vi "PumpCommand.vi"() -> ()   [LabVIEW 2022 SP3]
panel:
  in  "stop":bool
  in  "reference":refnum<visa-resource-name>
  in  "error in (no error)":errorcluster
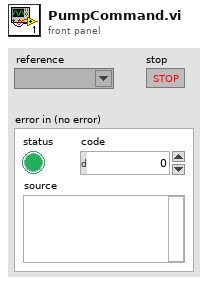
[diagram p1: front panel]
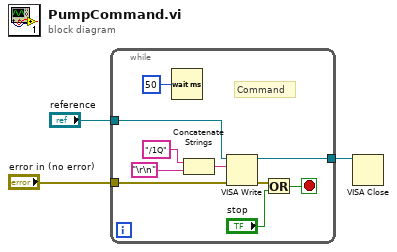
[diagram p0: block diagram]
diagram:
  n1 = while {
    tunnel: "error in (no error)" -> [w11]
    tunnel: "reference" -> [w10]
    tunnel: [w4] -> w1
    stop <- w5 stop-if-true
    # "Command"
    n2 = Wait (ms)(milliseconds to wait=u32 50) -> ()  [unwired: 1 out]
    n3 = Concatenate Strings("/1Q" ("write buffer"), "\r\n") -> (w9:string)
    n4 = VISA Write(VISA resource name=w10, write buffer=w9, error in (no error)=w11) -> (VISA resource name out=w4:refnum<visa-resource-name>, error out=w7:errorcluster)  [unwired: 1 out]
    n5 = Or(x=w7, y="stop") -> (x .or. y?=w5:bool)
  }
  n6 = VISA Close(VISA resource name=w1) -> ()  [unwired: 1 in, 1 out]
